vi "Perform Action.vi"(8 "error in":errorcluster, 10 "Input":variant, 11 "DO DAQmx Fixed Freq PWM CFG in":refnum<class "DO DAQmx Fixed Freq PWM CFG.lvclass">) -> (0 "error out":errorcluster, 2 "Output":variant, 3 "DO DAQmx Fixed Freq PWM CFG out":refnum<class "DO DAQmx Fixed Freq PWM CFG.lvclass">)   [LabVIEW 2023, in "DO DAQmx Fixed Freq PWM CFG.lvclass"]
uses:
  DO DAQmx Fixed Freq PWM CFG.lvclass
  DAQmx/DAQmx Base CFG/DAQmx Base CFG.lvclass/DAQmx Base CFG.ctl
  Configuration/Configuration Semaphore/CFG Semaphore.lvclass/CFG Semaphore.ctl
  DO DAQmx Fixed Freq PWM CFG.lvclass/DO DAQmx Fixed Freq PWM CFG.ctl
  <vilib>/DAQmx/write.llb/DAQmx Write (Digital 1D Wfm NChan NSamp).vi
  <vilib>/Waveform/DWDTOps.llb/DWDT Uncompress Digital.vi
  <vilib>/DAQmx/miscellaneous.llb/DAQmx Fill In Error Info.vi
  Configuration/Configuration Semaphore/CFG Semaphore.lvclass
  DAQmx/DAQmx Base CFG/DAQmx Base CFG.lvclass
  <userlib>/_OpenG.lib/time/time.llb/openg_time.lvlib
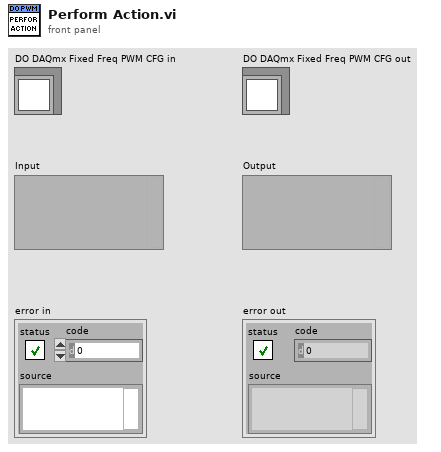
[diagram p1: front panel]
types:
  T1 = cluster{"Samplerate":dbl, "Samples per Channel":u32}
  T2 = cluster{"Channel":string, "Digital Waveform":digitalwaveform}[]
  T3 = cluster{"Channel":string, "digital waveform":digitalwaveform}
  T4 = typedef "Semaphore RefNum" = refnum<k1>
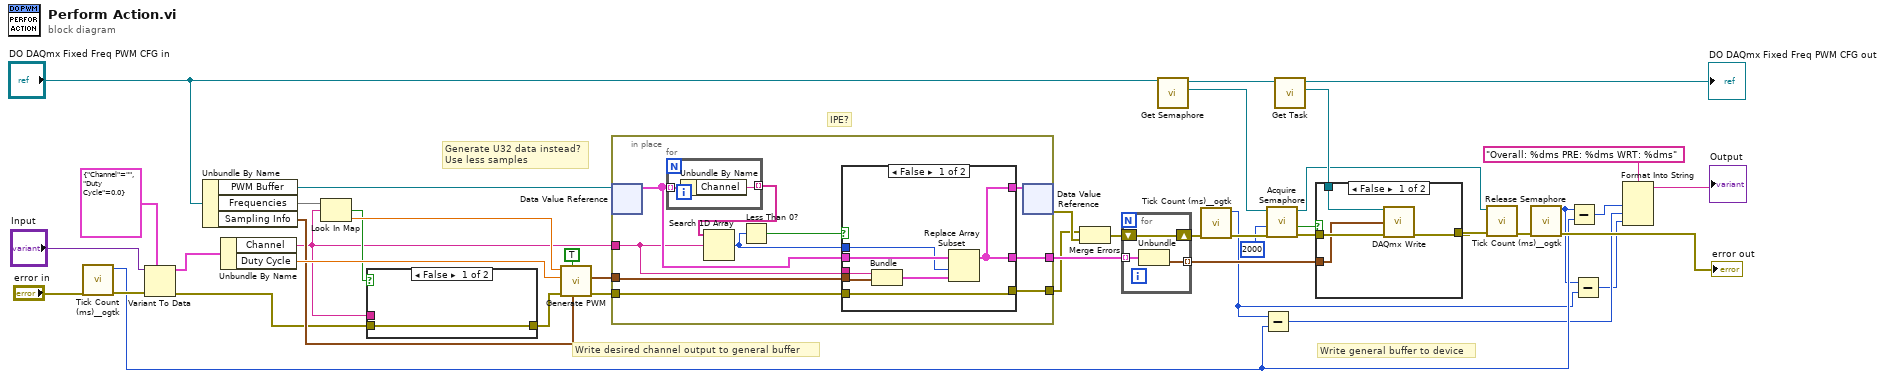
[diagram p0: block diagram]
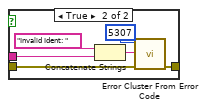
[diagram p2: hidden frame]
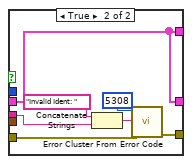
[diagram p3: hidden frame]
diagram:
  # "Generate U32 data instead?\nUse less samples"
  # "IPE?"
  # "Write general buffer to device"
  # "Write desired channel output to general buffer"
  n1 = call <userlib>:"Tick Count (ms)__ogtk.vi"("error in (no error)"="error in") -> ("error out"=w14:errorcluster, "millisecond timer value"=w10:u32)  [unwired: 9 in]
  n2 = Variant To Data(error in=w14, type=cluster{"Channel":string, "Duty Cycle":dbl} {"Channel"="", "Duty Cycle"=0.0}, Variant="Input") -> (data=w44:cluster{"Channel":string, "Duty Cycle":dbl}, error out=w21:errorcluster)
  n3 = Unbundle By Name("DO DAQmx Fixed Freq PWM CFG in") -> ("PWM Buffer"=w41:refnum<data-value>, "Frequencies"=w23:map{string, dbl}, "Sampling Info"=w24:T1)
  n4 = Unbundle By Name(w44) -> ("Channel"=w18:string, "Duty Cycle"=w33:dbl)
  n5 = Look In Map(map=w23, key=w18) -> (key not found?=w20:bool, value=w22:dbl)  [unwired: 1 in]
  n6 = case shown="False" w20 {
    tunnel: w21 -> [w45 w46]
    tunnel: [w45 w51] -> w19
    tunnel: w18 -> [_ w48]
    frame False {
    }
    frame True {
      n7 = Concatenate Strings("Invalid Ident: ", w48) -> (w50:string)
      n8 = call <vilib>:"Error Cluster From Error Code.vi"("error in (no error)"=w46, "error message (\"\")"=w50, "error code (0)"=5307) -> ("error out"=w51:errorcluster)  [unwired: 6 in]
    }
  }
  n9 = call "Generate PWM.vi"("sampling info"=w24, "reset?"=TRUE, "error in"=w19, "duty cycle"=w33, "frequency"=w22) -> ("error out"=w17:errorcluster, "digital waveform"=w40:digitalwaveform)  [unwired: 5 in]
  n10 = in-place {
    in-place-border: w18 -> [w55]
    in-place-border: w40 -> [w54]
    in-place-border: [w52] -> w32
    in-place-border: w17 -> [w58]
    in-place-border: [w57] -> w16
    n11 = in-place-dvr #1(w41) -> (w56:T2)  [unwired: 1 out]
    n12 = for {
      tunnel: w56 -> [w77] mode=indexing
      tunnel: [w76] -> w61 mode=indexing
      n13 = Unbundle By Name(w77) -> ("Channel"=w76:string)
    }
    n14 = Search 1D Array(1D array=w61, element=w55) -> (index of element=w59:i32)  [unwired: 1 in]
    n15 = Less Than 0?(x=w59) -> (x < 0?=w60:bool)
    n16 = case shown="False" w60 {
      tunnel: w59 -> [w66 _]
      tunnel: w58 -> [w68 w72]
      tunnel: [w68 w71] -> w57
      tunnel: w56 -> [w67 w69]
      tunnel: w55 -> [w65 w70]
      tunnel: w54 -> [w64 _]
      tunnel: [w62 w69] -> w53
      tunnel: [w62 w69] -> w52
      frame False {
        n17 = Bundle("Channel"=w65, "digital waveform"=w64) -> (w63:T3)  [unwired: 1 in]
        n18 = Replace Array Subset(array=w67, new element=w63, index=w66) -> (w62:T2)
      }
      frame True {
        n19 = Concatenate Strings("Invalid Ident: ", w70) -> (w75:string)
        n20 = call <vilib>:"Error Cluster From Error Code.vi"("error in (no error)"=w72, "error message (\"\")"=w75, "error code (0)"=5308) -> ("error out"=w71:errorcluster)  [unwired: 6 in]
      }
    }
    n21 = in-place-dvr #1(w53) -> (w30:errorcluster)  [unwired: 1 out]
  }
  n22 = Merge Errors(w16, w30) -> (w29:errorcluster)
  n23 = for {
    tunnel: w32 -> [w80] mode=indexing
    tunnel: [w79] -> w31 mode=indexing
    shift-right: [w78] -> w13
    shift-left: w29 -> [w78]
    n24 = Unbundle(w80) -> ("Digital Waveform"=w79:digitalwaveform)  [unwired: 1 out]
  }
  n25 = call "Get Semaphore.vi"("CFG Base in"="DO DAQmx Fixed Freq PWM CFG in") -> ("Semaphore"=w37:T4, "CFG Base out"=w38:refnum<class "DO DAQmx Fixed Freq PWM CFG.lvclass">)  [unwired: 9 in]
  n26 = call <userlib>:"Tick Count (ms)__ogtk.vi"("error in (no error)"=w13) -> ("error out"=w12:errorcluster, "millisecond timer value"=w5:u32)  [unwired: 9 in]
  n27 = Subtract(x=w5, y=w10) -> (x-y=w7:u32)
  n28 = call <vilib>:"Acquire Semaphore.vi"("error in (no error)"=w12, "ms timeout (-1)"=2000, "semaphore"=w37) -> ("error out"=w35:errorcluster, "timed out"=w36:bool, "semaphore out"=w27:T4)  [unwired: 2 in]
  n29 = call "Get Task.vi"("DAQmx Base CFG in"=w38) -> ("Task"=w34:refnum<k21>, "DAQmx Base CFG out"=→"DO DAQmx Fixed Freq PWM CFG out":refnum<class "DO DAQmx Fixed Freq PWM CFG.lvclass">)  [unwired: 9 in]
  n30 = case shown="False" w36 {
    tunnel: w35 -> [w83 w85]
    tunnel: w34 -> [w84 _]
    tunnel: w31 -> [w82 _]
    tunnel: [w81 w85] -> w28
    frame False {
      n31 = call-poly <vilib>:"DAQmx Write.vi"("task/channels in"=w84, "data"=w82, "error in"=w83) -> ("error out"=w81:errorcluster)  [unwired: 10 in, 2 out]
    }
    frame True {
    }
  }
  n32 = call <vilib>:"Release Semaphore.vi"("error in (no error)"=w28, "semaphore"=w27) -> ("error out"=w26:errorcluster)  [unwired: 4 in, 1 out]
  n33 = call <userlib>:"Tick Count (ms)__ogtk.vi"("error in (no error)"=w26) -> ("error out"=→"error out":errorcluster, "millisecond timer value"=w6:u32)  [unwired: 9 in]
  n34 = Subtract(x=w6, y=w10) -> (x-y=w8:u32)
  n35 = Subtract(x=w6, y=w5) -> (x-y=w4:u32)
  n36 = Format Into String(format string="Overall: %dms PRE: %dms WRT: %dms", w8, w7, w4) -> (resulting string=→"Output":string)  [unwired: 2 in, 1 out]
